vi "LV SciSDK TOF SPECTRUM RESET.vi"(8 "error in (no error)":errorcluster, 9 "Board Handle In":T1, 10 "TOF Spectrum Handle In":T2) -> (0 "error out":errorcluster, 1 "Board Handle Out":T1, 2 "TOF Spectrum Handle Out":T2, 3 "NI Error Code":i32)   [LabVIEW 2021, in "SciSDK_Labview.lvlib"]
doc: "You need this VI to execute 'reset' TOF spectrum component command"
uses:
  SciSDK_Labview.lvlib
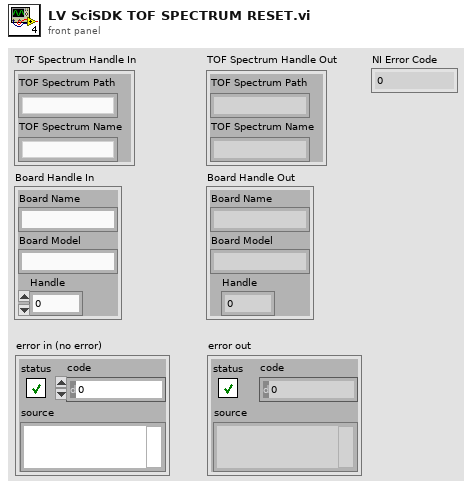
[diagram p1: front panel]
types:
  T1 = cluster{"Board Name":string, "Board Model":string, "Handle":u64}
  T2 = cluster{"TOF Spectrum Path":string, "TOF Spectrum Name":string}
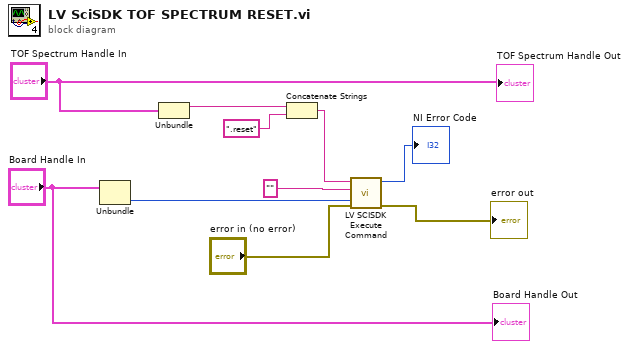
[diagram p0: block diagram]
diagram:
  n1 = Unbundle("Board Handle In") -> ("Handle"=w2:u64)  [unwired: 2 out]
  n2 = Unbundle("TOF Spectrum Handle In") -> ("TOF Spectrum Path"=w3:string)  [unwired: 1 out]
  n3 = Concatenate Strings(w3, ".reset" ("string")) -> (w8:string)
  n4 = call "LV SCISDK Execute Command.vi"("error in (no error)"="error in (no error)", "handle"=w2, "value"="", "Path"=w8) -> ("error out"=→"error out":errorcluster, "function return"=→"NI Error Code":i32)  [unwired: 5 in, 1 out]
  "TOF Spectrum Handle Out" <- "TOF Spectrum Handle In"
  "Board Handle Out" <- "Board Handle In"
